vi "JL_Continuous Cycle Mode Config.vi"(0 "GEA2 Reference In":refnum<k24>, 1 "Completed Cycles":u16, 2 "Enabled":u8, 5 "GEA Inputs":T1={"Source"=228, "Destination"=36} {"Destination" format="%.0x"; "Source" format="%.0x"}, 7 "TimeBetween Cycles":u32, 9 "Requested Cycles":u16, 11 "Error In":errorcluster) -> (4 "GEA2 Reference Out":refnum<k24>, 6 "Raw Data Out":string, 15 "Error Out":errorcluster)   [LabVIEW 2019]
uses:
  Common/LabVIEW GEA2 Toolkit/GEA3/type defs/Source_Destination.ctl
  D:/Common/LabVIEW GEA2 Toolkit/source/GEA3 DLL Source/GeaCommunication.dll
  Common/LabVIEW GEA2 Toolkit/source/GEA3 DLL Source/GeaCommunication.dll
  Common/LabVIEW GEA2 Toolkit/GEA3/type defs/ERD Write Data In.ctl
  Common/LabVIEW GEA2 Toolkit/GEA3/type defs/Data Type.ctl
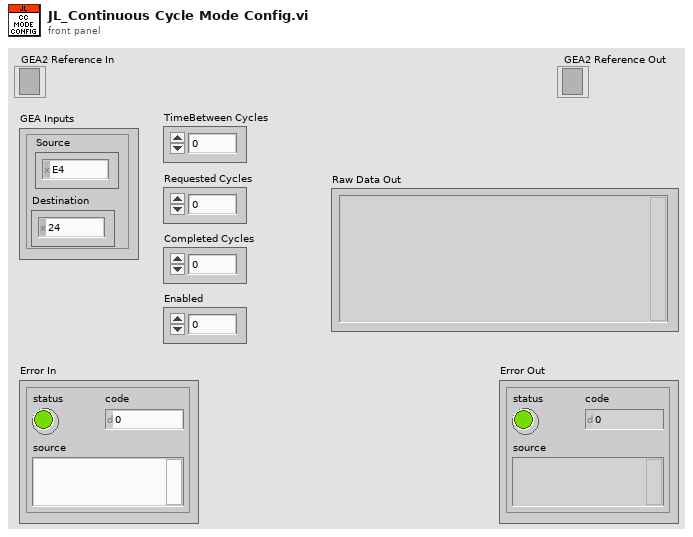
[diagram p1: front panel]
types:
  T1 = typedef "Source_Destination.ctl" = cluster{"Source":u8, "Destination":u8}
  T2 = typedef "ERD Write Data In.ctl" = cluster{"ERD Number":u16, "Data Type":T3, "Data":string}
  T3 = typedef "Data Type.ctl" = enum16{"string", "boolean", "uint8_t", "uint16_t", "uint32_t", "uint64_t", "int8_t", "int16_t", "int32_t", "int64_t"}
  T4 = cluster{"[0]":T2, "[1]":T2, "[2]":T2, "[3]":T2, "[4]":T2, "[5]":T2, "[6]":T2, "[7]":T2, "[8]":T2}
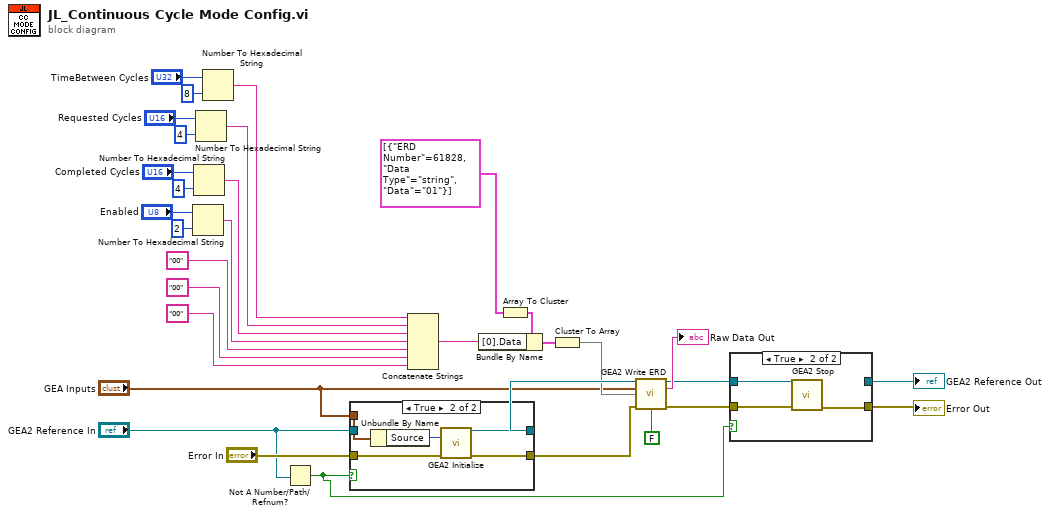
[diagram p0: block diagram]
diagram:
  n1 = Number To Hexadecimal String(1:i16 2 ("width (-)"), 2:"Enabled") -> (0:w28:string)
  n2 = Number To Hexadecimal String(1:i16 4 ("width (-)"), 2:"Completed Cycles") -> (0:w29:string)
  n3 = Number To Hexadecimal String(1:i16 4 ("width (-)"), 2:"Requested Cycles") -> (0:w30:string)
  n4 = Number To Hexadecimal String(1:i16 8 ("width (-)"), 2:"TimeBetween Cycles") -> (0:w31:string)
  n5 = Not A Number/Path/Refnum?(number/path/refnum="GEA2 Reference In") -> (NaN/Path/Refnum?=w2:bool)
  n6 = case shown="True" w2 {
    tunnel: "Error In" -> [w33 w39]
    tunnel: [w33 w38] -> w8
    tunnel: "GEA2 Reference In" -> [w34 _]
    tunnel: [w34 w37] -> w22
    tunnel: "GEA Inputs" -> [_ w35]
    frame False {
    }
    frame True {
      n7 = Unbundle By Name(w35) -> ("Source"=w36:u8)
      n8 = call "GEA2 Initialize.vi"("Source Address"=w36, "error in"=w39) -> ("GEA2 Reference Out"=w37:refnum<k24>, "error out"=w38:errorcluster)  [unwired: 11 in, 1 out]
    }
  }
  n9 = Concatenate Strings(w31, w30, w29, w28, "00" ("string"), "00" ("string"), "00" ("string")) -> (w26:string)
  n10 = Array To Cluster(array=T2[] [{"ERD Number"=61828, "Data Type"=enum."string", "Data"="01"}]) -> (cluster=w27:T4)
  n11 = Bundle By Name(cluster=w27, "[0].Data"=w26) -> (w32:T4)
  n12 = Cluster To Array(cluster=w32) -> (array=w21:T2[])
  n13 = call "GEA2 Write ERD.vi"("GEA2 Reference In"=w22, "GEA Inputs"="GEA Inputs", "Write ERD List"=w21, "Error In"=w8, "Verify ERD Response?"=FALSE) -> ("GEA2 Reference Out"=w10:refnum<k24>, "Raw Data Out"=→"Raw Data Out":string, "Error Out"=w9:errorcluster)  [unwired: 8 in]
  n14 = case shown="True" w2 {
    tunnel: w9 -> [w40 w43]
    tunnel: [w40 w42] -> w6
    tunnel: w10 -> [w41 w44]
    tunnel: [w41 _] -> w7
    frame False {
    }
    frame True {
      n15 = call "GEA2 Stop.vi"("GEA2 Reference In"=w44, "Error In"=w43) -> ("Error Out"=w42:errorcluster)  [unwired: 13 in]
    }
  }
  "GEA2 Reference Out" <- w7
  "Error Out" <- w6
